vi "TDMS Timestamp and Data.vi"(6 "channel name(s) in (Untitled)":string[](array[string]), 7 "timestamp":timestamp, 8 "error in (no error)":errorcluster, 9 "group name in (Untitled)":string, 10 "Array":dbl[](array[numeric]), 11 "Refnum in":refnum<k34>) -> (0 "error out":errorcluster, 3 "Refnum out":refnum<k34>)   [LabVIEW 2014]
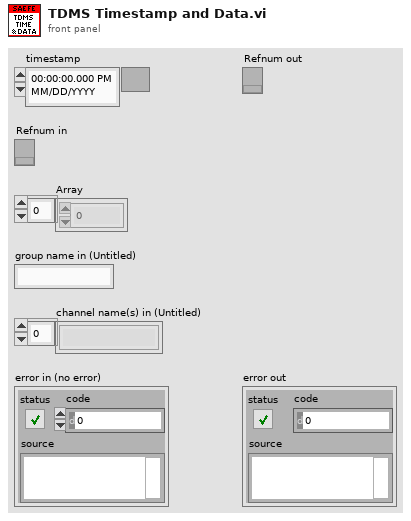
[diagram p1: front panel]
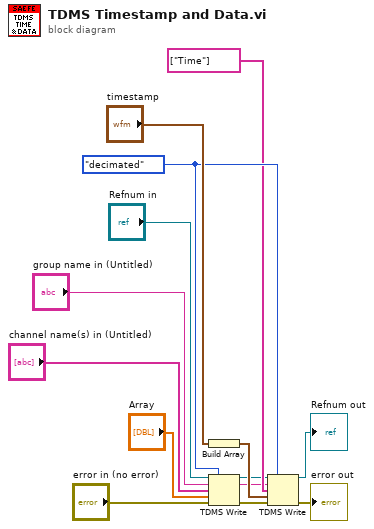
[diagram p0: block diagram]
diagram:
  w12 = enum16{"decimated", "interleaved"}."decimated" ("data layout (0:decimated)")
  n1 = Build Array("timestamp") -> (w14:timestamp[])
  n2 = TDMS Write(0:"Refnum in", 1:w12, 5:"group name in (Untitled)", 7:"channel name(s) in (Untitled)", 9:"Array", 11:"error in (no error)") -> (4:w5:refnum<k34>, 6:w9:string, 15:w6:errorcluster)  [unwired: 1 out]
  n3 = TDMS Write(0:w5, 1:w12, 5:w9, 7:string[] ["Time"] ("channel name(s) in (Untitled)"), 9:w14, 11:w6) -> (4:→"Refnum out":refnum<k34>, 15:→"error out":errorcluster)  [unwired: 2 out]
